vi "Toggle turn.vi"(8 "error in (no error)":errorcluster, 11 "Position in":refnum<class "Position.lvclass">) -> (0 "error out":errorcluster, 3 "Position out":refnum<class "Position.lvclass">)   [LabVIEW 2016, in "Chesslib.lvlib" / "Position.lvclass"]
uses:
  Position.lvclass
  Position.lvclass/Position.ctl
  typedef/Color.ctl
  Chesslib.lvlib
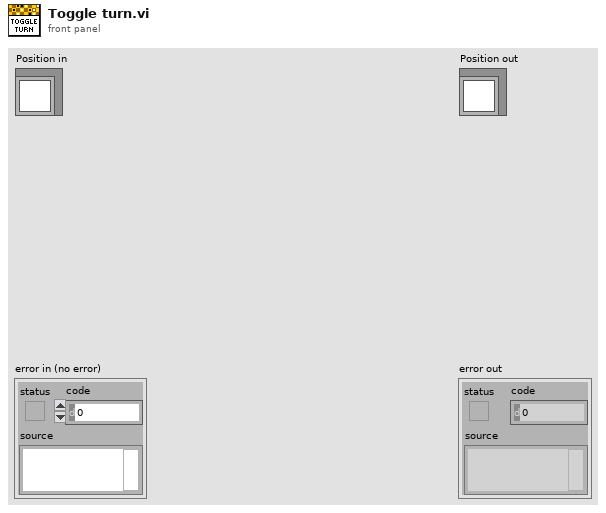
[diagram p1: front panel]
types:
  T1 = typedef "Chesslib.lvlib/Color.ctl" = enum16{"White", "Black"}
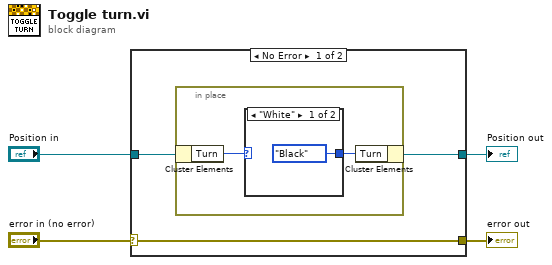
[diagram p0: block diagram]
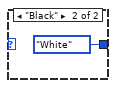
[diagram p2: hidden frame]
diagram:
  n1 = case shown="No Error" "error in (no error)" {
    selector: "error in (no error)" -> [w7 w13]
    tunnel: [w7 w13] -> w3
    tunnel: [w5 w12] -> w1
    tunnel: "Position in" -> [w6 w12]
    frame No Error {
      n2 = in-place {
        n3 = in-place-cluster #1(w6) -> ("Turn"=w9:T1)
        n4 = case shown="\"White\"" w9 {
          tunnel: [Color."Black" ("Turn") Color."White" ("Turn")] -> w8
          frame "White" {
          }
          frame "Black" {
          }
        }
        n5 = in-place-cluster #1("Turn"=w8) -> (w5:refnum<class "Position.lvclass">)
      }
    }
    frame Error {
    }
  }
  "error out" <- w3
  "Position out" <- w1
